vi "Error log.vi"(7 "File Ops":T1(ring), 8 "error in (no error)":errorcluster, 10 "Call Chain":string[](array[string]), 11 "time stamp":timestamp) -> (0 "error out 2":errorcluster)   [LabVIEW 2020]
panel:
  out "folder names":string[](array[string])
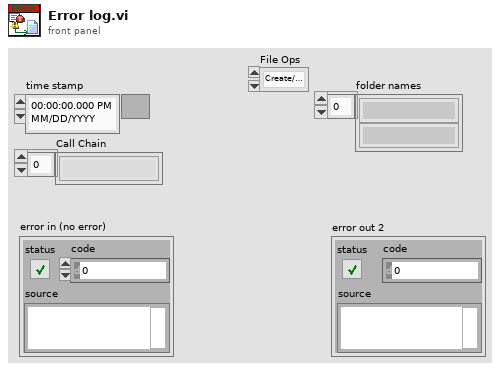
[diagram p1: front panel]
types:
  T1 = enum16{"Create/Open File", "Write File", "Close file"}
  T2 = enum16{"open", "replace", "create", "open or create", "replace or create", "replace or create with confirmation"}
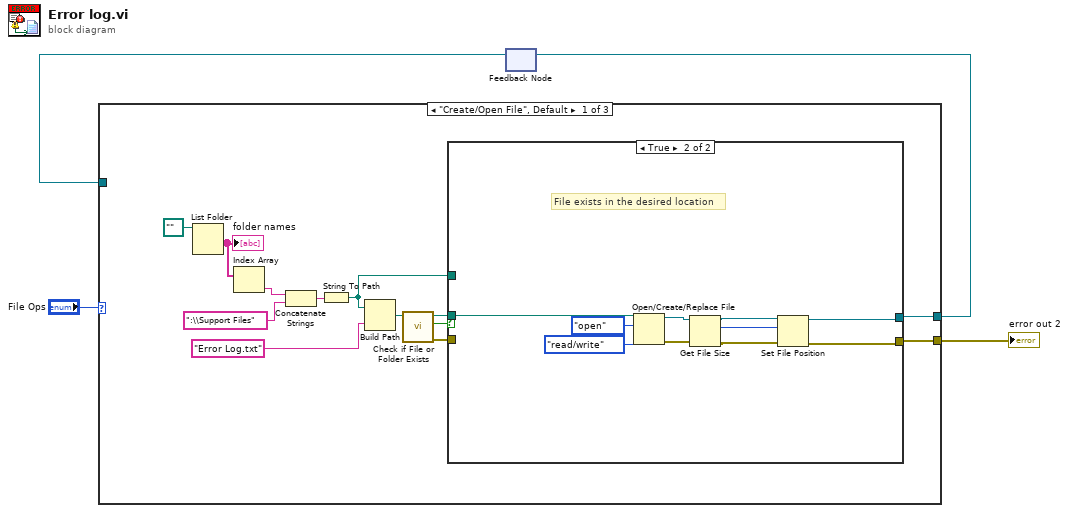
[diagram p0: block diagram]
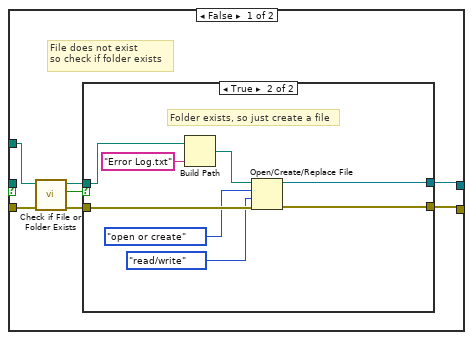
[diagram p2: hidden frame]
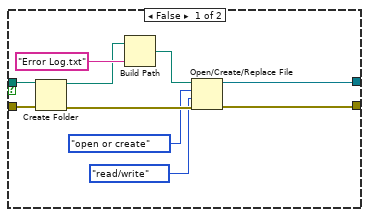
[diagram p3: hidden frame]
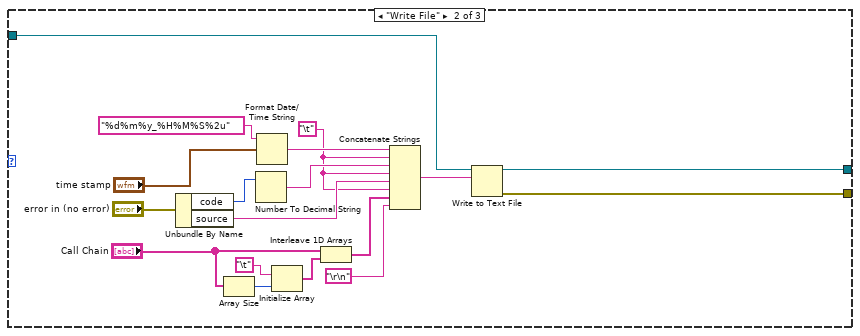
[diagram p4: hidden frame]
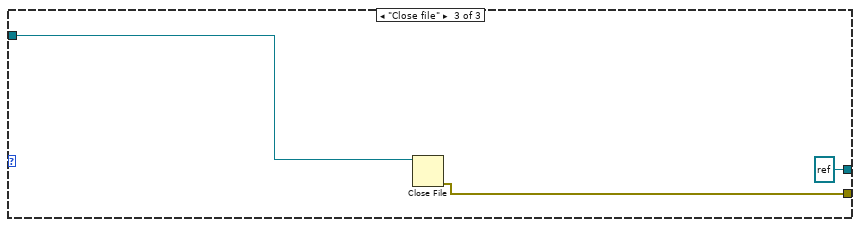
[diagram p5: hidden frame]
diagram:
  n1 = feedback #1() -> (w1:refnum<file>)  [unwired: 1 in]
  n2 = case shown="\"Create/Open File\", Default" "File Ops" {
    tunnel: [w9 w54 w71] -> w3
    tunnel: [w8 w53 refnum<file> refnum ("refnum out")] -> w2
    tunnel: w1 -> [_ w56 w73]
    frame "Create/Open File", Default {
      n3 = List Folder(path=path "") -> (folder names=w17:string[])  [unwired: 3 in, 3 out]
      "folder names" <- w17
      n4 = Index Array(array=w17) -> (element=w16:string)  [unwired: 1 in]
      n5 = Concatenate Strings(w16, ":\\Support Files" ("string")) -> (w15:string)
      n6 = String To Path(string=w15) -> (path=w6:path)
      n7 = Build Path(base path=w6, name or relative path="Error Log.txt") -> (appended path=w14:path)
      n8 = call <vilib>:"Check if File or Folder Exists.vi"("path"=w14) -> ("error out"=w5:errorcluster, "file or folder exists?"=w11:bool, "dup path"=w10:path)  [unwired: 8 in]
      n9 = case shown="True" w11 {
        tunnel: w10 -> [_ w52]
        tunnel: [w18 w48] -> w9
        tunnel: [w19 w49] -> w8
        tunnel: w6 -> [w21 _]
        tunnel: w5 -> [w24 _]
        frame False {
          # "File does not exist\nso check if folder exists"
          n10 = call <vilib>:"Check if File or Folder Exists.vi"("error in (no error)"=w24, "path"=w21) -> ("error out"=w23:errorcluster, "file or folder exists?"=w22:bool, "dup path"=w20:path)  [unwired: 7 in]
          n11 = case shown="True" w22 {
            tunnel: w23 -> [w34 w39]
            tunnel: w20 -> [w33 w41]
            tunnel: [w27 w37] -> w19
            tunnel: [w28 w38] -> w18
            frame False {
              n12 = Create Folder(path (use dialog)=w33, error in=w34) -> (created path=w29:path, error out=w30:errorcluster)  [unwired: 1 in, 1 out]
              n13 = Build Path(base path=w29, name or relative path="Error Log.txt") -> (appended path=w31:path)
              n14 = Open/Create/Replace File(file path (use dialog)=w31, error in=w30, operation (0:open)=T2."open or create", access (0:read/write)=enum16{"read/write", "read-only", "write-only"}."read/write") -> (refnum out=w27:refnum<file>, error out=w28:errorcluster)  [unwired: 2 in, 1 out]
            }
            frame True {
              # "Folder exists, so just create a file"
              n15 = Build Path(base path=w41, name or relative path="Error Log.txt") -> (appended path=w40:path)
              n16 = Open/Create/Replace File(file path (use dialog)=w40, error in=w39, operation (0:open)=T2."open or create", access (0:read/write)=enum16{"read/write", "read-only", "write-only"}."read/write") -> (refnum out=w37:refnum<file>, error out=w38:errorcluster)  [unwired: 2 in, 1 out]
            }
          }
        }
        frame True {
          # "File exists in the desired location"
          n17 = Open/Create/Replace File(file path (use dialog)=w52, operation (0:open)=T2."open", access (0:read/write)=enum16{"read/write", "read-only", "write-only"}."read/write") -> (refnum out=w46:refnum<file>, error out=w47:errorcluster)  [unwired: 3 in, 1 out]
          n18 = Get File Size(file=w46, error in=w47) -> (refnum out=w45:refnum<file>, size (in bytes)=w43:i64, 0:w44:errorcluster)
          n19 = Set File Position(offset (in bytes) (0)=w43, refnum=w45, error in=w44) -> (refnum out=w49:refnum<file>, error out=w48:errorcluster)  [unwired: 1 in]
        }
      }
    }
    frame "Write File" {
      w62 = "\t"
      n20 = Unbundle By Name("error in (no error)") -> ("code"=w69:i32, "source"=w67:string)
      n21 = Array Size(array="Call Chain") -> (size(s)=w66:i32)
      n22 = Number To Decimal String(number=w69) -> (decimal integer string=w68:string)  [unwired: 1 in]
      n23 = Format Date/Time String(time format string (%c)="%d%m%y_%H%M%S%2u", seconds (now)="time stamp") -> (date/time string=w70:string)  [unwired: 1 in]
      n24 = Initialize Array("\t", w66) -> (w65:string[])
      n25 = Interleave 1D Arrays("Call Chain", w65) -> (w64:string[])
      n26 = Concatenate Strings(w70, w62, w68, w62, w67, w62, w64, "\r\n") -> (w55:string)
      n27 = Write to Text File(file (use dialog)=w56, text=w55) -> (refnum out=w53:refnum<file>, error out=w54:errorcluster)  [unwired: 2 in, 1 out]
    }
    frame "Close file" {
      n28 = Close File(refnum=w73) -> (error out=w71:errorcluster)  [unwired: 1 in, 1 out]
    }
  }
  "error out 2" <- w3
  n29 = feedback-in #1(w2) -> ()
